vi "Get_Amount_Displacement_in_Column-1.vi"(2 "multiplier":i32=4, 3 "# Rows":i32) -> (0 "multiplier out":i32=4, 1 "Displ amount":i32)   [LabVIEW 2017]
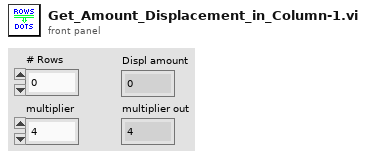
[diagram p1: front panel]
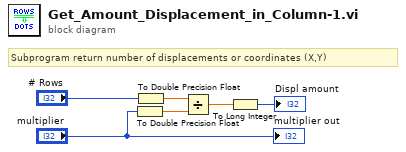
[diagram p0: block diagram]
diagram:
  # "Subprogram return number of displacements or coordinates (X,Y)"
  n1 = To Double Precision Float(number="multiplier") -> (double precision float=w3:dbl)
  n2 = To Double Precision Float(number="# Rows") -> (double precision float=w1:dbl)
  n3 = Divide(x=w1, y=w3) -> (x/y=w6:dbl)
  n4 = To Long Integer(number=w6) -> (32bit integer=→"Displ amount":i32)
  "multiplier out" <- "multiplier"
